vi "SineOrSawtooth.vi"(3 "error in (no error)":errorcluster, 4 "Parameters":T2={"number of planes"=4, "z step"=1.9999999999999998e-05, "pixel dwell time"=1.0000000000000001e-11, "z frequency"=10.0, "number of pixels"=100, "smooth points"=10, "smooth line"=10, "Sine\nSawtooth"=FALSE, "PointSorting"=0, "Sort Points"=FALSE, "X-pixels"=256.0, "Y-lines"=256.0, "pixelstoµm"=256.0, "zoom"=1.0, "Time offset"=1.0000000000000001e-11} {"zoom" min=0.5 step=0.1; "Y-lines" min=1 step=1; "X-pixels" min=1 step=1; "PointSorting" items=["No Difference", "Every Second Point", "Down / Up"]; "smooth line" min=1; "smooth points" min=1; "number of pixels" min=1; "z frequency" format="%_4g"; "number of planes" min=1}, 5 "DutyCluster":T1 {"Iteration" items=["first iteration", "second iteration"]}) -> (0 "error out":errorcluster, 1 "DutyCluster":T1 {"Iteration" items=["first iteration", "second iteration"]})   [LabVIEW 2010]
uses:
  TypeDefs/DutyCluster.ctl
  TypeDefs/ParameterCluster.ctl
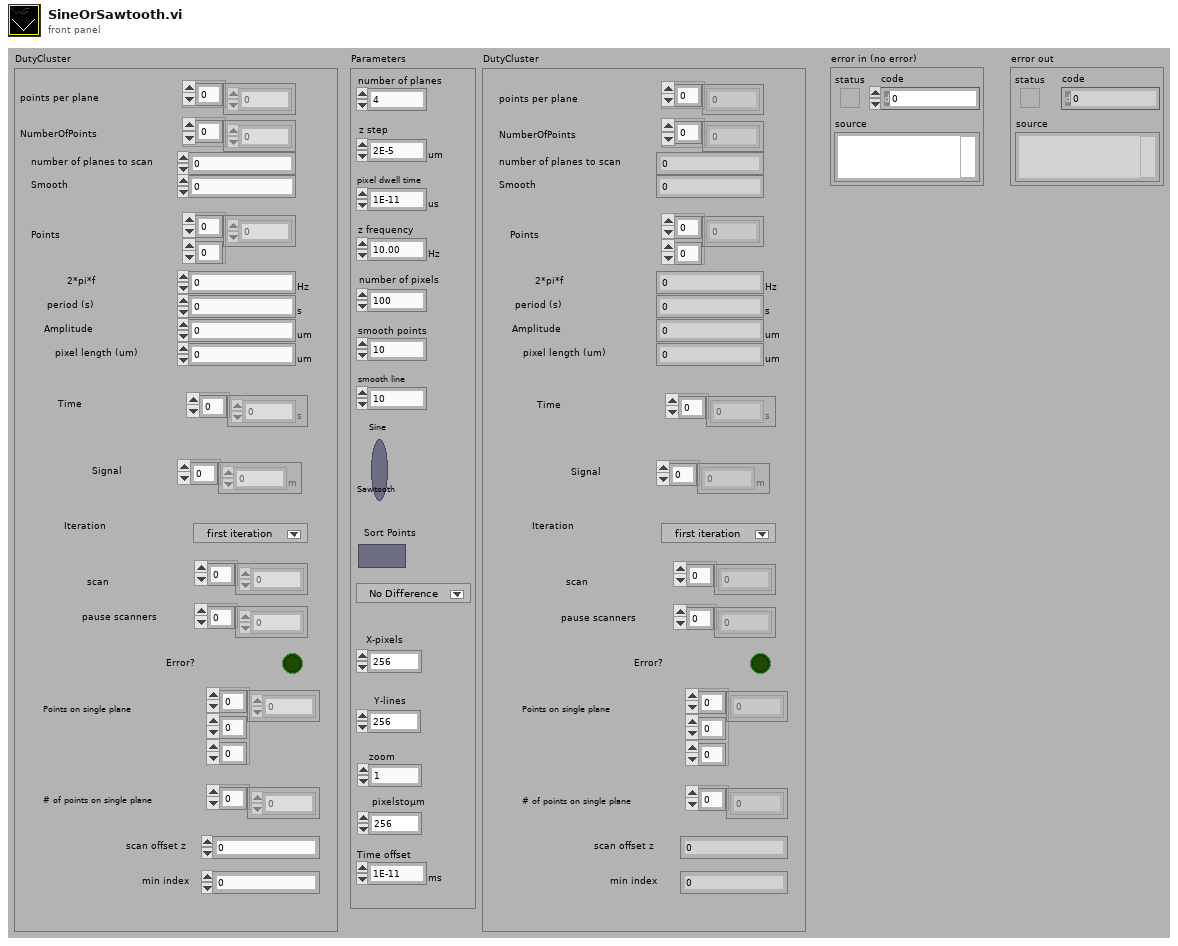
[diagram p1: front panel]
types:
  T1 = typedef "DutyCluster.ctl" = cluster{"points per plane":i32[], "NumberOfPoints":i32[], "number of planes to scan":i32, "Smooth":i32, "Points":dbl[][], "2*pi*f":dbl[unit], "period (s)":dbl[unit], "Amplitude":dbl[unit], "pixel length (um)":dbl[unit], "Time":dbl[unit][], "Signal":dbl[unit][], "Iteration":u16, "scan":i32[], "pause scanners":i32[], "Error?":bool, "Points on single plane":dbl[][][], "# of points on single plane":i32[], "scan offset z":i32, "min index":i32}
  T2 = typedef "ParameterCluster.ctl" = cluster{"number of planes":i32, "z step":dbl[unit], "pixel dwell time":dbl[unit], "z frequency":dbl[unit], "number of pixels":i32, "smooth points":i32, "smooth line":i32, "Sine\nSawtooth":bool, "PointSorting":u16, "Sort Points":bool, "X-pixels":sgl, "Y-lines":sgl, "pixelstoµm":dbl, "zoom":dbl, "Time offset":dbl[unit]}
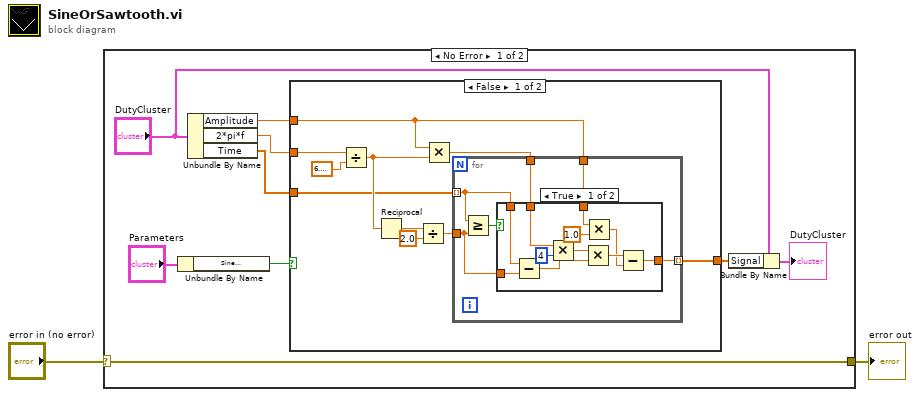
[diagram p0: block diagram]
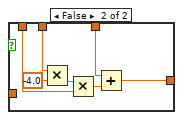
[diagram p2: hidden frame]
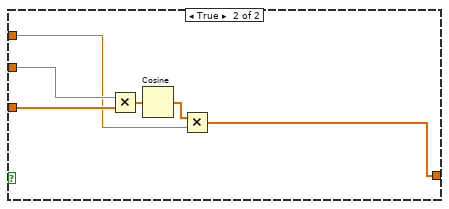
[diagram p3: hidden frame]
diagram:
  n1 = case shown="No Error" "error in (no error)" {
    selector: "error in (no error)" -> [w7 w52]
    tunnel: [w7 w52] -> w1
    frame No Error {
      n2 = Unbundle By Name("Parameters") -> ("Sine\nSawtooth"=w8:bool)
      n3 = Unbundle By Name("DutyCluster") -> ("Amplitude"=w11:dbl[unit], "2*pi*f"=w10:dbl[unit], "Time"=w6:dbl[unit][])
      n4 = case shown="False" w8 {
        tunnel: w11 -> [w20 w47]
        tunnel: w10 -> [w18 w49]
        tunnel: w6 -> [w13 w48]
        tunnel: [w12 w46] -> w4
        frame False {
          n5 = Divide(x=w18, y=6.283185307179586) -> (x/y=w14:dbl[unit])
          n6 = Reciprocal(x=w14) -> (1/x=w17:dbl[unit])
          n7 = Divide(x=w17, y=2.0) -> (x/y=w15:dbl[unit])
          n8 = Multiply(x=w20, y=w14) -> (x*y=w21:dbl[unit])
          n9 = for {
            tunnel: w21 -> [w24]
            tunnel: w13 -> [w23] mode=indexing
            tunnel: w20 -> [w26]
            tunnel: w15 -> [w22]
            tunnel: [w25] -> w12 mode=indexing
            n10 = Greater Or Equal?(x=w23, y=w22) -> (x >= y?=w27:bool)
            n11 = case shown="True" w27 {
              tunnel: w23 -> [w28 w39]
              tunnel: w26 -> [w31 w42]
              tunnel: [w34 w41] -> w25
              tunnel: w24 -> [w36 w40]
              tunnel: w22 -> [w30 _]
              frame True {
                n12 = Subtract(x=w28, y=w30) -> (x-y=w29:dbl[unit])
                n13 = Multiply(x=w36, y=4) -> (x*y=w38:dbl[unit])
                n14 = Multiply(x=w38, y=w29) -> (x*y=w35:dbl[unit])
                n15 = Multiply(x=w31, y=1.0) -> (x*y=w32:dbl[unit])
                n16 = Subtract(x=w35, y=w32) -> (x-y=w34:dbl[unit])
              }
              frame False {
                n17 = Multiply(x=w40, y=-4.0) -> (x*y=w45:dbl[unit])
                n18 = Multiply(x=w45, y=w39) -> (x*y=w44:dbl[unit])
                n19 = Add(x=w42, y=w44) -> (x+y=w41:dbl[unit])
              }
            }
          }
        }
        frame True {
          n20 = Multiply(x=w49, y=w48) -> (x*y=w51:dbl[])
          n21 = Cosine(x=w51) -> (cos(x)=w50:dbl[])
          n22 = Multiply(x=w50, y=w47) -> (x*y=w46:dbl[unit][])
        }
      }
      n23 = Bundle By Name(cluster="DutyCluster", "Signal"=w4) -> (→"DutyCluster":T1)
    }
    frame Error {
    }
  }
  "error out" <- w1
